vi "Cycle Angle to Crank U16 and Cycle Count.vi"(10 "rotations":u16, 11 "cycle angle":dbl) -> (1 "degrees of one u16":dbl, 2 "cycle count":fxp<+,2,2>, 3 "crank U16":u16)   [LabVIEW 2017, in "Engine Simulation Toolkit System Explorer.lvlib"]
uses:
  Engine Simulation Toolkit System Explorer.lvlib
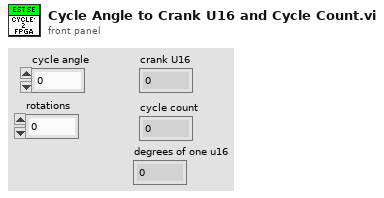
[diagram p1: front panel]
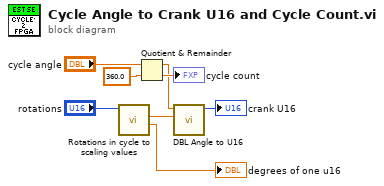
[diagram p0: block diagram]
diagram:
  n1 = call "Rotations in cycle to scaling values.vi"("rotations in a cycle"="rotations") -> ("degrees of one u16"=→"degrees of one u16":dbl, "angle to u16 scale factor"=w8:dbl)  [unwired: 8 in, 1 out]
  n2 = Quotient & Remainder(x="cycle angle", y=360.0 ("t")) -> (x-y*floor(x/y)=w3:dbl, floor(x/y)=→"cycle count":dbl)
  n3 = call "DBL Angle to U16.vi"("angle to u16 scale factor"=w8, "Desired angle (degrees)"=w3) -> ("u16"=→"crank U16":u16)  [unwired: 8 in, 1 out]
